vi "Write Cam Attr 2 ini file.vi"(8 "error in (no error)":errorcluster, 9 "Appl Params":variant, 10 "refnum in":T1, 11 "IMAQdx Cam in":refnum<class "IMAQdx Cam.lvclass">) -> (0 "error out":errorcluster, 1 "Appl Params out":variant, 2 "refnum out":T1, 3 "IMAQdx Cam out":refnum<class "IMAQdx Cam.lvclass">)   [LabVIEW 2014, in "IMAQdx Cam.lvclass"]
doc: "VI reads attributes filter from viariant Appl Parameters: property \"Cam attribute filters\" of type string array. E.g. for a Balser scout GigE camera filter \"Exposure\" would select all attributes including string \"exposure\" case insensitive:\n\nCamera Attributes::Acquisition Controls::Exposure Time (Abs) = 1,852000E+3\nCamera Attributes::Acquisition Controls::Exposure Timebase = 1,000000E+0\nCamera Attributes::Acquisition Controls::Enable Exposure Timebase = TRUE\n....\n\nFrom variant property \"Cam dont save attributes\" of type string array VI reads attributes to ve excluded from storage.\ne.g. \"Enable Exposure Timebase\" would remove last entry:\n\nCamera Attributes::Acquisition Controls::Exposure Time (Abs) = 1,852000E+3\nCamera Attributes::Acquisition Controls::Exposure Timebase = 1,000000E+0\n\nIf these variant properties are not set, VI use defoult filter: Exposure, Shutter, Gain, and exclusion filter: Bayer, Evet, Limit.\n\n--------------\nauthor: Alexander Kessler, Helmholtz-Institut-Jena \nmaintainer: Alexander Kessler: alexander.kessler@uni-jena.de\n\n\n\nLicense Agreement for this software:\n\nCopyright (C)\nHelmholtz-Institut-Jena\nFröbelstieg 3\n07743 Jena\nGermany\n\nThis program is free software; you can redistribute it and/or modify it under the terms of the GNU General Public License as published by the Free Software Foundation; either version 2 of the license, or (at your option) any later version.\n\nThis program is distributed in the hope that it will be useful, but WITHOUT ANY WARRANTY; without even the implied warranty of MERCHANTABILITY or FITNESS FOR A PARTICULAR PURPOSE. See the GNU General License for more details (http://www.gnu.org)."
uses:
  IMAQdx Cam.lvclass
  <vilib>/Utility/config.llb/Config Data RefNum.ctl
  <vilib>/Utility/config.llb/NI_LVConfig.lvlib
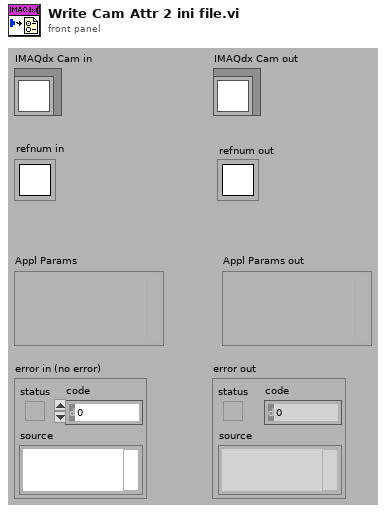
[diagram p1: front panel]
types:
  T1 = typedef "NI_LVConfig.lvlib/Config Data RefNum.ctl" = refnum<k1>
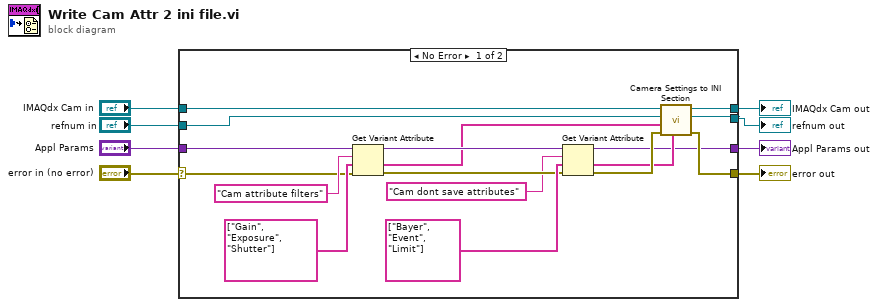
[diagram p0: block diagram]
diagram:
  n1 = case shown="No Error" "error in (no error)" {
    selector: "error in (no error)" -> [w22 w29]
    tunnel: [w14 w29] -> w7
    tunnel: [w20 w28] -> w5
    tunnel: "IMAQdx Cam in" -> [w21 w28]
    tunnel: "Appl Params" -> [w25 w26]
    tunnel: "refnum in" -> [w11 w27]
    tunnel: [w10 w27] -> w2
    tunnel: [w9 w26] -> w1
    frame No Error {
      n2 = Get Variant Attribute(Variant=w25, name="Cam attribute filters", default value (empty Variant)=string[] ["Gain", "Exposure", "Shutter"] ("Filters"), error in=w22) -> (duplicate Variant=w18:variant, value=w12:string[], error out=w17:errorcluster)  [unwired: 1 out]
      n3 = Get Variant Attribute(Variant=w18, name="Cam dont save attributes", default value (empty Variant)=string[] ["Bayer", "Event", "Limit"] ("do not save"), error in=w17) -> (duplicate Variant=w9:variant, value=w13:string[], error out=w15:errorcluster)  [unwired: 1 out]
      n4 = call-dynamic "Camera Settings to INI Section.vi"("do not save"=w13, "error in (no error)"=w15, "Filters"=w12, "refnum in"=w11, "IMAQdx Cam in"=w21) -> ("error out"=w14:errorcluster, "refnum out"=w10:T1, "IMAQdx Cam out"=w20:refnum<class "IMAQdx Cam.lvclass">)  [unwired: 4 in]
    }
    frame Error {
    }
  }
  "error out" <- w7
  "IMAQdx Cam out" <- w5
  "refnum out" <- w2
  "Appl Params out" <- w1
